vi "2283_girarGrados.vi"(1 "gyro":cluster{"angle":dbl, "anglerate":dbl}, 2 "angulo deseado":dbl) -> (0 "g output":dbl(slide) scale=-1.0..1.0)   [LabVIEW 2014]
uses:
  <vilib>/addons/control/pid/pid.llb/PID (DBL).vi
  <vilib>/addons/control/pid/NI_PID_pid.lvlib
panel:
  out "upper limit":dbl
  in  "PID gains":T1={"proportional gain (Kc)"=1.0, "integral time (Ti, min)"=0.01, "derivative time (Td, min)"=0.0} {"derivative time (Td, min)" format="%.3f"; "integral time (Ti, min)" format="%.3f"; "proportional gain (Kc)" format="%.3f"}
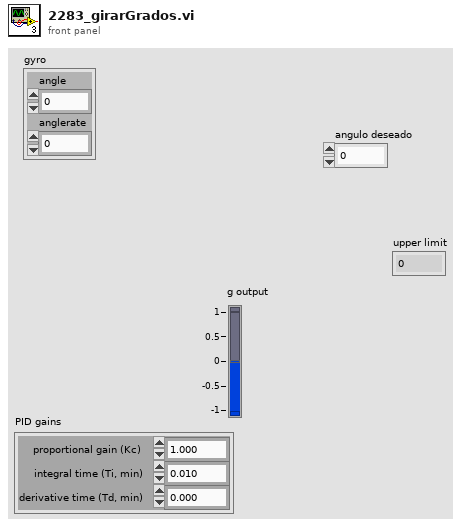
[diagram p1: front panel]
types:
  T1 = cluster{"proportional gain (Kc)":dbl, "integral time (Ti, min)":dbl, "derivative time (Td, min)":dbl}
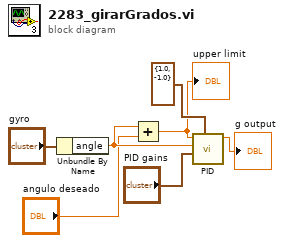
[diagram p0: block diagram]
diagram:
  n1 = Unbundle By Name("gyro") -> ("angle"=w4:dbl)
  n2 = Add(x=w4, y="angulo deseado") -> (x+y=w3:dbl)
  "upper limit" <- w3
  n3 = call-poly <vilib>:"PID.vi"("output range"=cluster{"output high":dbl, "output low":dbl} {"output high"=1.0, "output low"=-1.0}, "PID gains"="PID gains", "process variable"=w4, "setpoint"=w3) -> ("output"=→"g output":dbl)  [unwired: 6 in, 1 out]
